vi "Create System Output References.vi"(8 "error in (no error)":errorcluster, 11 "Device Item Ref in":T1 format="%.0x") -> (0 "error out":errorcluster)   [LabVIEW 2020, in "G5 Regatron Custom Device System Explorer.lvlib"]
uses:
  G5 Regatron Custom Device System Explorer.lvlib
  <vilib>/NI VeriStand/Custom Device API/Custom Device Channel Type.ctl
  <vilib>/NI VeriStand/Custom Device API/Custom Device API.lvlib
  <vilib>/NI VeriStand/Custom Device API/Custom Device Channel.ctl
  <vilib>/NI VeriStand/Custom Device API/Custom Device Item Ref.ctl
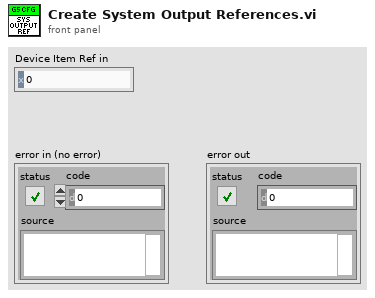
[diagram p1: front panel]
types:
  T1 = typedef "Custom Device API.lvlib/Custom Device Item Ref.ctl" = u64
  T2 = typedef "Custom Device API.lvlib/Custom Device Channel.ctl" = cluster{"Type":T3, "Units":string, "Default Value":dbl, "Faultable":bool, "Scalable":bool}
  T3 = typedef "Custom Device API.lvlib/Custom Device Channel Type.ctl" = enum16{"Input", "Output"}
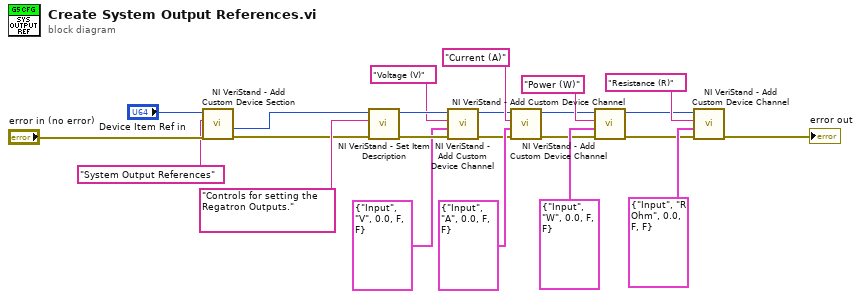
[diagram p0: block diagram]
diagram:
  n1 = call <vilib>:"NI VeriStand - Add Custom Device Section.vi"("error in (no error)"="error in (no error)", "Section Name"="System Output References", "Parent Ref in"="Device Item Ref in") -> ("error out"=w19:errorcluster, "Section Ptr"=w21:T1)  [unwired: 5 in, 2 out]
  n2 = call <vilib>:"NI VeriStand - Set Item Description.vi"("error in (no error)"=w19, "Description"="Controls for setting the Regatron Outputs.", "Item Ref in"=w21) -> ("error out"=w20:errorcluster, "Item Ref out"=w22:T1)  [unwired: 6 in, 1 out]
  n3 = call <vilib>:"NI VeriStand - Add Custom Device Channel.vi"("error in (no error)"=w20, "Channel"=T2 {"Type"=enum."Input", "Units"="V", "Default Value"=0.0, "Faultable"=FALSE, "Scalable"=FALSE}, "Channel Name"="Voltage (V)", "Parent Ref in"=w22) -> ("error out"=w3:errorcluster, "Parent Ref out"=w4:T1)  [unwired: 4 in, 2 out]
  n4 = call <vilib>:"NI VeriStand - Add Custom Device Channel.vi"("error in (no error)"=w3, "Channel"=T2 {"Type"=enum."Input", "Units"="A", "Default Value"=0.0, "Faultable"=FALSE, "Scalable"=FALSE}, "Channel Name"="Current (A)", "Parent Ref in"=w4) -> ("error out"=w5:errorcluster, "Parent Ref out"=w6:T1)  [unwired: 4 in, 2 out]
  n5 = call <vilib>:"NI VeriStand - Add Custom Device Channel.vi"("error in (no error)"=w5, "Channel"=T2 {"Type"=enum."Input", "Units"="W", "Default Value"=0.0, "Faultable"=FALSE, "Scalable"=FALSE}, "Channel Name"="Power (W)", "Parent Ref in"=w6) -> ("error out"=w8:errorcluster, "Parent Ref out"=w9:T1)  [unwired: 4 in, 2 out]
  n6 = call <vilib>:"NI VeriStand - Add Custom Device Channel.vi"("error in (no error)"=w8, "Channel"=T2 {"Type"=enum."Input", "Units"="R Ohm", "Default Value"=0.0, "Faultable"=FALSE, "Scalable"=FALSE}, "Channel Name"="Resistance (R)", "Parent Ref in"=w9) -> ("error out"=→"error out":errorcluster)  [unwired: 4 in, 3 out]
